vi "MyGlobal.vi"() -> ()   [LabVIEW 2018]
uses:
  SwerveDrive.ctl
  Drivetype.ctl
  Face Avant.ctl
panel:
  in  "Disque relache":bool
  in  "Face Avant":T1
  in  "Auto Disque":bool
  in  "Auto R Trigger":dbl
  in  "Auto L Trigger":dbl
  in  "Auto axe Y":dbl
  in  "Auto axe X":dbl
  in  "Roue en place":bool
  in  "Autonome":bool
  in  "Assenceur bas":bool
  in  "Assenceur haut":bool
  in  "Boussole":dbl
  in  "Boussole init":dbl
  in  "Correction angle":dbl
  in  "potentiometre":dbl
  in  "Direction Ascenseur":dbl=-1.0
  in  "POV":dbl
  in  "L Trigger":dbl
  in  "R Trigger":dbl
  in  "Ascenseur":dbl
  in  "X-Disque":bool
  in  "Position Reel Ascenseur":u8
  in  "Etage Ascenseur Previous":u8
  in  "Potentiometre Valeurs Etages":dbl[](array[numeric])=[0.0, 1.0, 2.0, 3.0, 4.0, 5.0]
  in  "type mouvement":T2=enum."1 vitesse"
  in  "Etage Ascenseur":u8
  in  "A - Ramasse Ballon":bool
  in  "B - Lance Ballon":bool
  in  "SwerveDrive":T3
  in  "Axe R X":dbl
  in  "Axe R Y":dbl
  in  "angle arriere gauche":dbl
  in  "angle arriere droit":dbl
  in  "angle avant gauche":dbl
  in  "Vitesse robot":dbl
  in  "FinMouvements":bool
  in  "angle avant droit":dbl
  in  "Bouton 4":bool
  in  "Bouton 2":bool
  in  "Bouton 3":bool
  in  "RB - Disque":bool
  in  "Bouton 5":bool
  in  "Bouton 1":bool
  in  "axe z":dbl
  in  "axe y":dbl
  in  "axe x":dbl
  in  "Hello":dbl
  # "Global Data"
  # "Joystick 2 - Co Pilot"
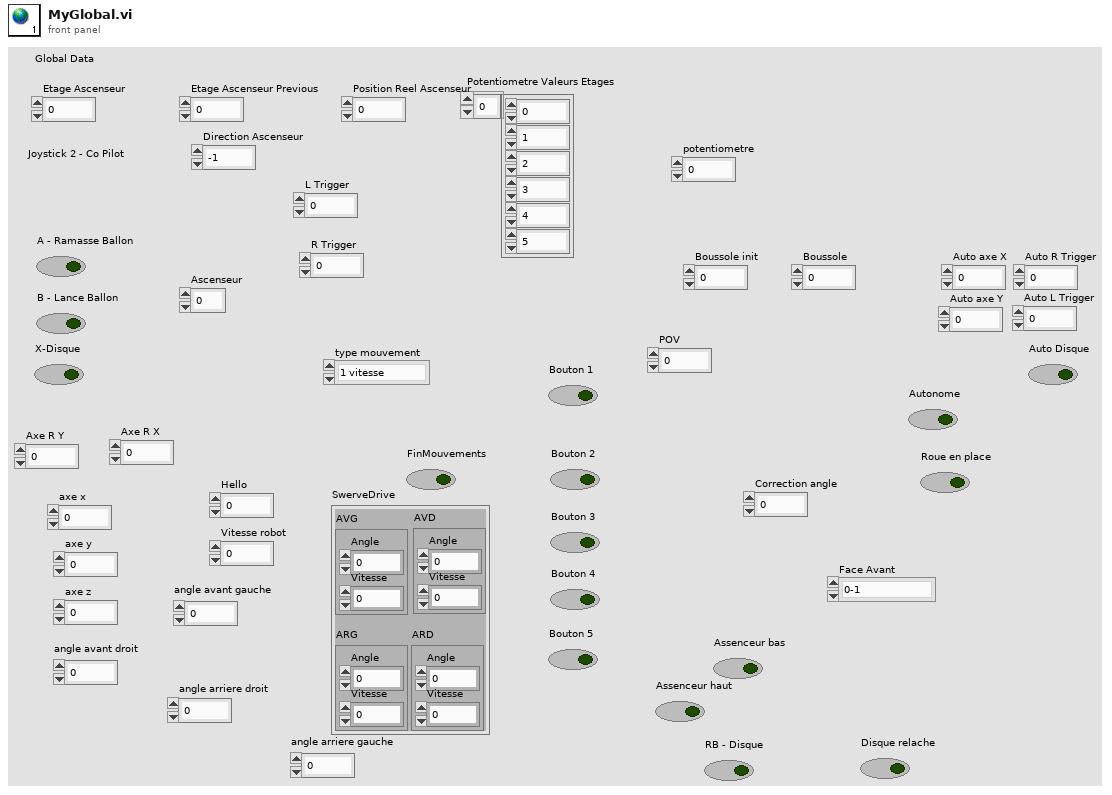
[diagram p1: front panel]
types:
  T1 = typedef "Face Avant.ctl" = enum16{"0-1", "1-2", "2-3", "3-0"}
  T2 = typedef "Drivetype.ctl" = enum16{"4 vitesse", "1 vitesse"}
  T3 = typedef "SwerveDrive.ctl" = cluster{"AVD":cluster{"Angle":dbl, "Vitesse":dbl}, "AVG":cluster{"Angle":dbl, "Vitesse":dbl}, "ARG":cluster{"Angle":dbl, "Vitesse":dbl}, "ARD":cluster{"Angle":dbl, "Vitesse":dbl}}
diagram:
